vi "calcule_heure_jour_nuit.vi"(2 "Tableau fin":timestamp[](array[timestamp]), 3 "Tableau debut":timestamp[](array[timestamp])) -> (0 "nombre heures nuit":dbl, 1 "nombre heures jour":dbl)   [LabVIEW 2024]
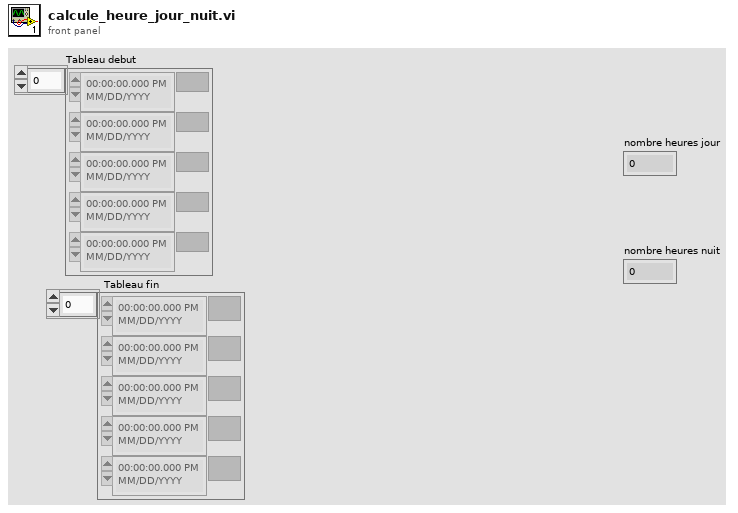
[diagram p1: front panel]
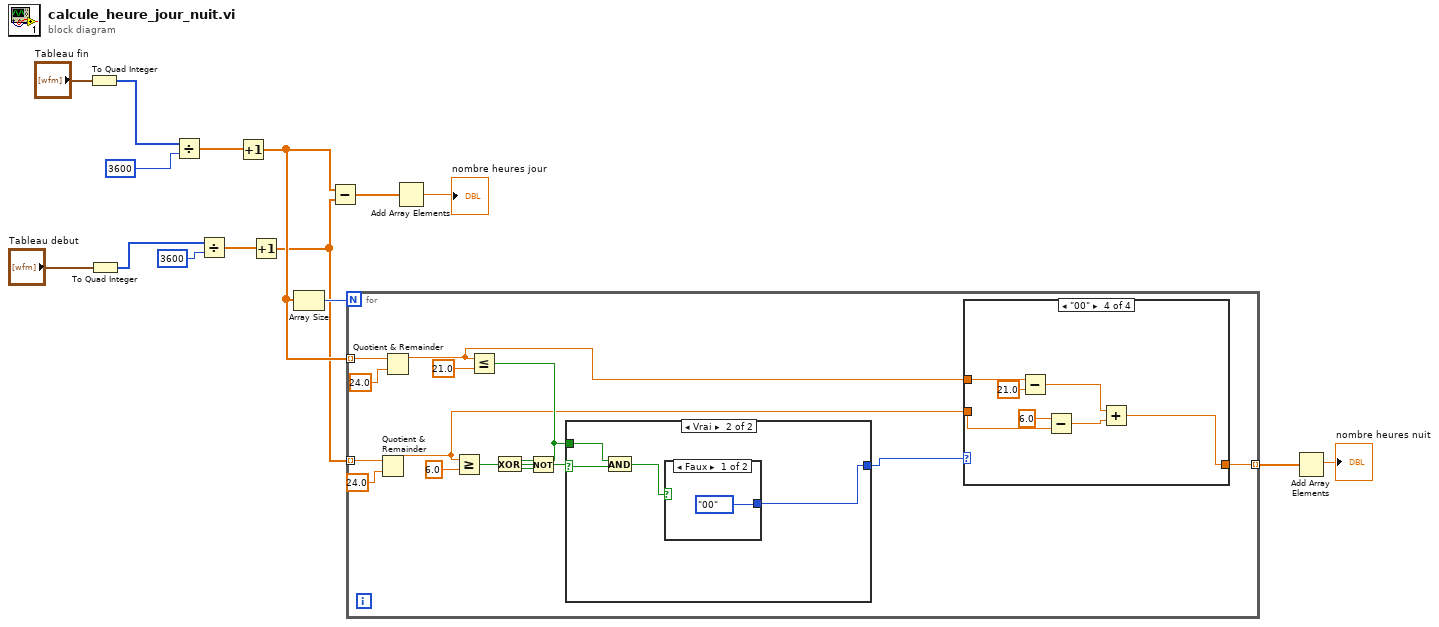
[diagram p0: block diagram]
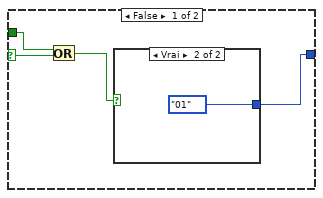
[diagram p2: hidden frame]
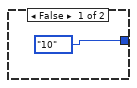
[diagram p3: hidden frame]
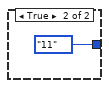
[diagram p4: hidden frame]
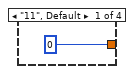
[diagram p5: hidden frame]
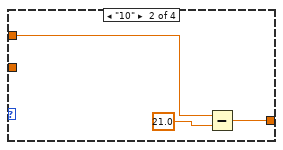
[diagram p6: hidden frame]
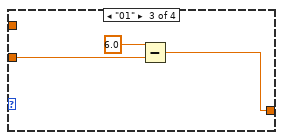
[diagram p7: hidden frame]
diagram:
  n1 = To Quad Integer(1:"Tableau fin") -> (0:w12:i64[])
  n2 = To Quad Integer(1:"Tableau debut") -> (0:w10:i64[])
  n3 = Divide(x=w12, y=3600) -> (x/y=w9:dbl[])
  n4 = Divide(x=w10, y=3600) -> (x/y=w7:dbl[])
  n5 = Increment(x=w9) -> (x+1=w6:dbl[])
  n6 = Increment(x=w7) -> (x+1=w5:dbl[])
  n7 = Array Size(array=w6) -> (size(s)=w8:i32)
  n8 = Subtract(x=w6, y=w5) -> (x-y=w3:dbl[])
  n9 = for {
    N: w8 -> [_]
    tunnel: [w29] -> w2 mode=indexing
    tunnel: w6 -> [w19] mode=indexing
    tunnel: w5 -> [w18] mode=indexing
    n10 = Quotient & Remainder(x=w18, y=24.0) -> (x-y*floor(x/y)=w17:dbl)  [unwired: 1 out]
    n11 = Quotient & Remainder(x=w19, y=24.0) -> (x-y*floor(x/y)=w16:dbl)  [unwired: 1 out]
    n12 = Greater Or Equal?(x=w17, y=6.0) -> (x >= y?=w25:bool)
    n13 = Less Or Equal?(x=w16, y=21.0) -> (x <= y?=w24:bool)
    n14 = Exclusive Or(1:w25, 2:w24) -> (0:w23:bool)
    n15 = Not(x=w23) -> (.not. x?=w22:bool)
    n16 = case shown="Vrai" w22 {
      selector: w22 -> [w32 w38]
      tunnel: [w31 w37] -> w26
      tunnel: w24 -> [w33 w39]
      frame False {
        n17 = Or(x=w33, y=w32) -> (x .or. y?=w30:bool)
        n18 = case shown="Vrai" w30 {
          tunnel: [enum16{"11", "10", "01", "00"}."10" enum16{"11", "10", "01", "00"}."01"] -> w31
          frame False {
          }
          frame True {
          }
        }
      }
      frame True {
        n19 = And(x=w39, y=w38) -> (x .and. y?=w36:bool)
        n20 = case shown="Faux" w36 {
          tunnel: [enum16{"11", "10", "01", "00"}."00" enum16{"11", "10", "01", "00"}."11"] -> w37
          frame False {
          }
          frame True {
          }
        }
      }
    }
    n21 = case shown="\"00\"" w26 {
      tunnel: [0 w43 w46 w53] -> w29
      tunnel: w16 -> [_ w44 _ w51]
      tunnel: w17 -> [_ _ w48 w49]
      frame "11", Default {
      }
      frame "10" {
        n22 = Subtract(x=w44, y=21.0) -> (x-y=w43:dbl)
      }
      frame "01" {
        n23 = Subtract(x=6.0, y=w48) -> (x-y=w46:dbl)
      }
      frame "00" {
        n24 = Subtract(x=w51, y=21.0) -> (x-y=w55:dbl)
        n25 = Subtract(x=6.0, y=w49) -> (x-y=w54:dbl)
        n26 = Add(x=w55, y=w54) -> (x+y=w53:dbl)
      }
    }
  }
  n27 = Add Array Elements(numeric array=w3) -> (sum=→"nombre heures jour":dbl)
  n28 = Add Array Elements(numeric array=w2) -> (sum=→"nombre heures nuit":dbl)
